vi "MAIN PROVVISORIO.vi"() -> ()   [LabVIEW 2019]
uses:
  <vilib>/DAQmx/configure/timing.llb/DAQmx Timing (Sample Clock).vi
  <vilib>/DAQmx/create/channels.llb/DAQmx Create Channel (CI-Count Edges).vi
  <vilib>/DAQmx/read.llb/DAQmx Read (Counter 1D U32 1Chan NSamp).vi
  <vilib>/DAQmx/read.llb/DAQmx Read (Analog 1D Wfm NChan NSamp).vi
  <vilib>/DAQmx/read.llb/DAQmx Read (Counter 1D DBL 1Chan NSamp).vi
  <vilib>/DAQmx/create/channels.llb/DAQmx Create Channel (AI-Voltage-Basic).vi
  <vilib>/DAQmx/create/channels.llb/DAQmx Create Channel (CI-Frequency).vi
  <vilib>/DAQmx/configure/timing.llb/DAQmx Timing (Implicit).vi
  <vilib>/Analysis/NI_AALBase.lvlib
  <vilib>/Analysis/baseanly.llb/Mean (DBL).vi
  <resource>/objmgr/daqmx.rc
  TypeDef/MISURE WT.ctl
panel:
  in  "divisor":u32=4
  in  "Tab Control":T1(tab)
  out "MISURE DA WATTMETRO":T2
  out "Waveform Chart":waveform(dbl)[](graph)
  in  "Pause Button":bool
  out "x-y":u32
  out "size(s)":i32
  in  "Initial Count":u32(ring)
  in  "Count Direction":i32(ring)=10128 items=["Count Up"=10128, "Count Down"=10124, "Externally Controlled"=10326]
  in  "Edge":i32(ring)=10280 items=["Rising"=10280, "Falling"=10171]
  in  "Analog Channel":tag="MOMENTIVEMod2/ai0:1"
  in  "Counter Input - Frequency":tag="MOMENTIVEMod1/ctr0"
  in  "Counter Input - Count Edges":tag="MOMENTIVEMod1/ctr2"
  in  "Counter Input - Count Edges Terminal":tag="/MOMENTIVEMod1/PFI0"
  in  "CI.Freq.Term":tag="/MOMENTIVEMod1/PFI1"
  in  "Rate":dbl=10000.0 format="%0.2f"
  in  "Samples per channel":i32=2000
  out "error out":errorcluster
  out "error out 2":errorcluster
  out "error out 3":errorcluster
  out "error out 4":errorcluster
  out "error out 5":errorcluster
  out "error out 6":errorcluster
  in  "Fondoscala NM":dbl=500.0
  out "COPPIA [NM]":dbl
  out "Speed [RPM]":dbl format="%#.6f"
  out "P[kW]":dbl
  in  "OFFSET NM":dbl
  in  "stop":bool
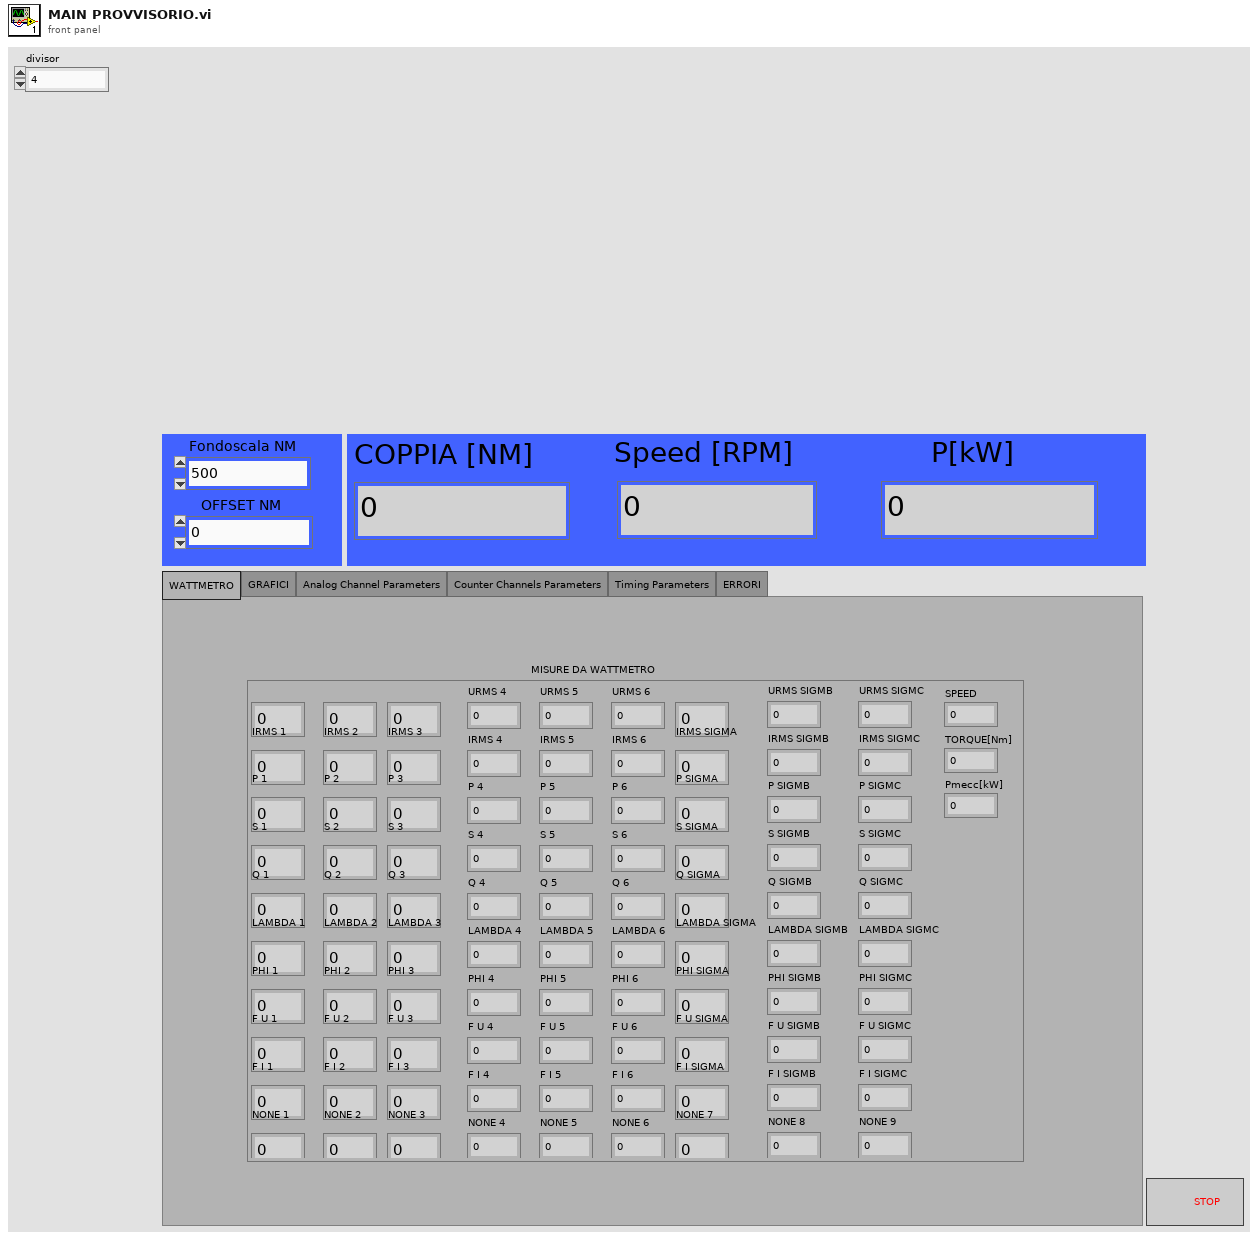
[diagram p1: front panel]
types:
  T1 = enum32{"WATTMETRO", "GRAFICI", "Analog Channel Parameters", "Counter Channels Parameters", "Timing Parameters", "ERRORI"}
  T2 = typedef "MISURE WT.ctl" = cluster{"URMS 1":dbl, "IRMS 1":dbl, "P 1":dbl, "S 1":dbl, "Q 1":dbl, "LAMBDA 1":dbl, "PHI 1":dbl, "F U 1":dbl, "F I 1":dbl, "NONE 1":dbl, "URMS 2":dbl, "IRMS 2":dbl, "P 2":dbl, "S 2":dbl, "Q 2":dbl, "LAMBDA 2":dbl, "PHI 2":dbl, "F U 2":dbl, "F I 2":dbl, "NONE 2":dbl, "URMS 3":dbl, "IRMS 3":dbl, "P 3":dbl, "S 3":dbl, "Q 3":dbl, "LAMBDA 3":dbl, "PHI 3":dbl, "F U 3":dbl, "F I 3":dbl, "NONE 3":dbl, "URMS 4":dbl, "IRMS 4":dbl, "P 4":dbl, "S 4":dbl, "Q 4":dbl, "LAMBDA 4":dbl, "PHI 4":dbl, "F U 4":dbl, "F I 4":dbl, "NONE 4":dbl, "URMS 5":dbl, "IRMS 5":dbl, "P 5":dbl, "S 5":dbl, "Q 5":dbl, "LAMBDA 5":dbl, "PHI 5":dbl, "F U 5":dbl, "F I 5":dbl, "NONE 5":dbl, "URMS 6":dbl, "IRMS 6":dbl, "P 6":dbl, "S 6":dbl, "Q 6":dbl, "LAMBDA 6":dbl, "PHI 6":dbl, "F U 6":dbl, "F I 6":dbl, "NONE 6":dbl, "URMS SIGMA":dbl, "IRMS SIGMA":dbl, "P SIGMA":dbl, "S SIGMA":dbl, "Q SIGMA":dbl, "LAMBDA SIGMA":dbl, "PHI SIGMA":dbl, "F U SIGMA":dbl, "F I SIGMA":dbl, "NONE 7":dbl, "URMS SIGMB":dbl, "IRMS SIGMB":dbl, "P SIGMB":dbl, "S SIGMB":dbl, "Q SIGMB":dbl, "LAMBDA SIGMB":dbl, "PHI SIGMB":dbl, "F U SIGMB":dbl, "F I SIGMB":dbl, "NONE 8":dbl, "URMS SIGMC":dbl, "IRMS SIGMC":dbl, "P SIGMC":dbl, "S SIGMC":dbl, "Q SIGMC":dbl, "LAMBDA SIGMC":dbl, "PHI SIGMC":dbl, "F U SIGMC":dbl, "F I SIGMC":dbl, "NONE 9":dbl, "SPEED":dbl, "TORQUE[Nm]":dbl, "Pmecc[kW]":dbl}
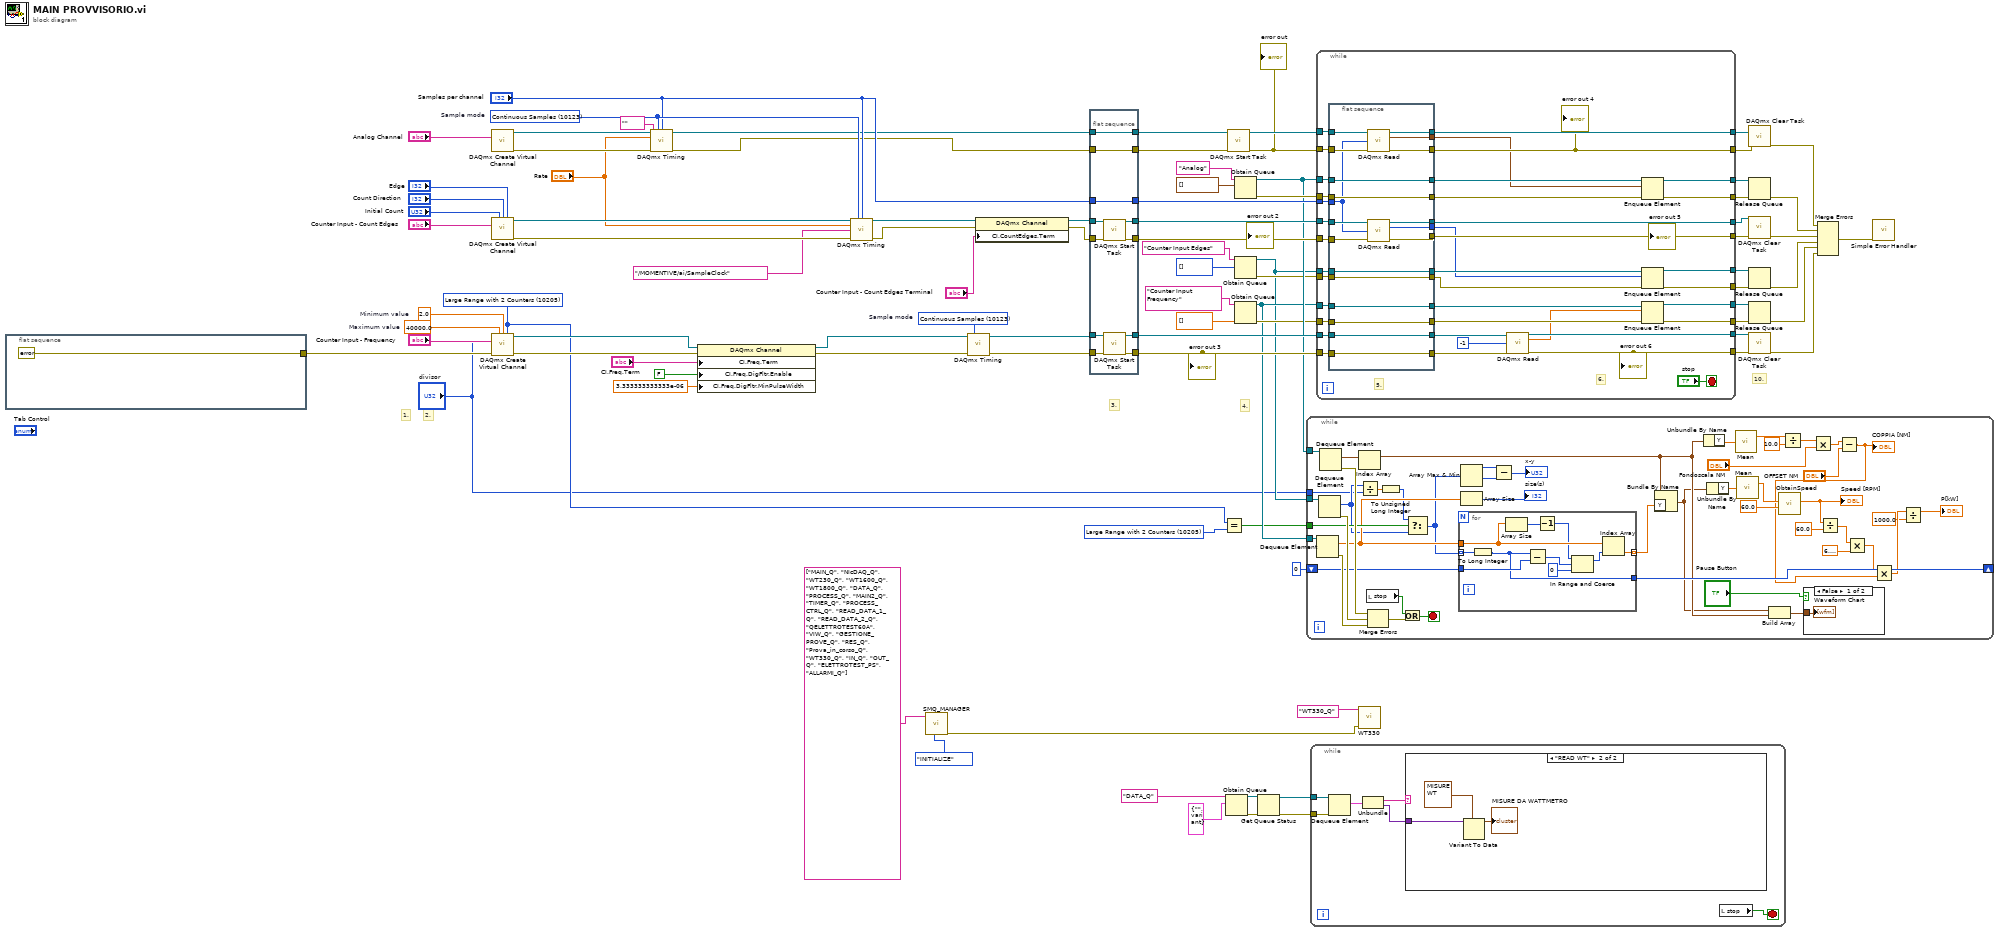
[diagram p0: block diagram]
diagram:
  w13 = 10205 items=["Low Frequency with 1 Counter"=10105, "High Frequency with 2 Counters"=10157, "Large Range with 2 Counters"=10205, "Dynamic Averaging"=16065] ("measurement method")
  w14 = 10205 items=["Low Frequency with 1 Counter"=10105, "High Frequency with 2 Counters"=10157, "Large Range with 2 Counters"=10205, "Dynamic Averaging"=16065] ("measurement method")
  w59 = 40000.0  # Maximum value
  w58 = 2.0  # Minimum value
  w60 = 10123 items=["Finite Samples"=10178, "Continuous Samples"=10123, "Hardware Timed Single Point"=12522]  # Sample mode
  w72 = 10123 items=["Finite Samples"=10178, "Continuous Samples"=10123, "Hardware Timed Single Point"=12522]  # Sample mode
  # "10."
  # "4."
  # "3."
  # "2."
  # "1."
  n1 = flat-sequence {
    tunnel: [errorcluster {"status"=FALSE, "code"=0, "source"=""} ("error constant")] -> w30
    frame #0 {
    }
  }
  n2 = call-poly <vilib>:"DAQmx Create Virtual Channel.vi"("physical channels"="Analog Channel") -> ("task out"=w83:refnum<k21>, "error out"=w82:errorcluster)  [unwired: 8 in, 5 out]
  n3 = call-poly <vilib>:"DAQmx Create Virtual Channel.vi"("initial count"="Initial Count", "count direction"="Count Direction", "edge"="Edge", "counter"="Counter Input - Count Edges") -> ("task out"=w84:refnum<k21>, "error out"=w76:errorcluster)  [unwired: 3 in, 7 out]
  n4 = call-poly <vilib>:"DAQmx Create Virtual Channel.vi"("maximum value"=w59, "minimum value"=w58, "measurement method"=w14, "counter"="Counter Input - Frequency", "divisor"="divisor", "error in"=w30) -> ("task out"=w23:refnum<k21>, "error out"=w21:errorcluster)  [unwired: 6 in, 2 out]
  n5 = call-poly <vilib>:"DAQmx Timing.vi"("task/channels in"=w83, "sample mode"=w72, "samples per channel"="Samples per channel", "rate"="Rate", "source"=tag "", "error in"=w82) -> ("task out"=w16:refnum<k21>, "error out"=w18:errorcluster)  [unwired: 1 in, 7 out]
  n6 = property class="DAQmx Channel"(reference=w23, error in=w21, "CI.Freq.Term"="CI.Freq.Term", "CI.Freq.DigFltr.Enable"=FALSE ("DI.DigFltr.Enable"), "CI.Freq.DigFltr.MinPulseWidth"=3.333333333333e-06 ("DI.DigFltr.MinPulseWidth")) -> (reference out=w22:refnum<k21>, error out=w20:errorcluster)
  n7 = call-poly <vilib>:"DAQmx Timing.vi"("task/channels in"=w84, "sample mode"=w72, "samples per channel"="Samples per channel", "rate"="Rate", "source"=tag "/MOMENTIVE/ai/SampleClock", "error in"=w76) -> ("task out"=w29:refnum<k21>, "error out"=w68:errorcluster)  [unwired: 1 in, 7 out]
  n8 = call <userlib>:"SMQ_MANAGER.vi"("Function"=enum16{"INITIALIZE", "ENQUEUE", "STOP ALL"}."INITIALIZE", "Queue array"=string[] ["MAIN_Q", "NIcDAQ_Q", "WT230_Q", "WT1600_Q", "WT1800_Q", "DATA_Q", "PROCESS_Q", "MAIN2_Q", "TIMER_Q", "PROCESS_CTRL_Q", "READ_DATA_1_Q", "READ_DATA_2_Q", "QELETTROTEST60A", "VIW_Q", "GESTIONE_PROVE_Q", "RES_Q", "Prova_in_corso_Q", "WT330_Q", "IN_Q", "OUT_Q", "ELETTROTEST_PS", "ALLARMI_Q"]) -> ("error out"=w7:errorcluster)  [unwired: 9 in]
  n9 = call-poly <vilib>:"DAQmx Timing.vi"("task/channels in"=w22, "sample mode"=w60, "error in"=w20) -> ("task out"=w27:refnum<k21>, "error out"=w28:errorcluster)  [unwired: 4 in, 7 out]
  n10 = property class="DAQmx Channel"(reference=w29, error in=w68, "CI.CountEdges.Term"="Counter Input - Count Edges Terminal") -> (reference out=w70:refnum<k21>, error out=w69:errorcluster)
  n11 = flat-sequence {
    tunnel: [w102] -> w75
    tunnel: [w101] -> w71
    tunnel: w70 -> [w100]
    tunnel: w69 -> [w99]
    tunnel: w27 -> [w98]
    tunnel: w28 -> [w97]
    tunnel: w16 -> [w96]
    tunnel: [w96] -> w66
    tunnel: [w95] -> w65
    tunnel: w18 -> [w95]
    tunnel: [w94] -> w64
    tunnel: [w93] -> w63
    tunnel: "Samples per channel" -> [w92]
    tunnel: [w92] -> w55
    frame #0 {
      n12 = call <vilib>:"DAQmx Start Task.vi"("task/channels in"=w100, "error in"=w99) -> ("task out"=w102:refnum<k21>, "error out"=w101:errorcluster)  [unwired: 12 out]
      n13 = call <vilib>:"DAQmx Start Task.vi"("task/channels in"=w98, "error in"=w97) -> ("task out"=w94:refnum<k21>, "error out"=w93:errorcluster)  [unwired: 12 out]
    }
  }
  n14 = Equal?(x=w14, y=w13) -> (x = y?=w12:bool)
  n15 = Obtain Queue(name (unnamed)="DATA_Q" ("Queue Name"), element data type=cluster{"String":string, "variant":variant} {"String"="", "variant"=variant} ("element")) -> (queue out=w4:refnum<queue>, error out=w3:errorcluster)  [unwired: 3 in, 1 out]
  n16 = call <vilib>:"DAQmx Start Task.vi"("task/channels in"=w66, "error in"=w65) -> ("task out"=w81:refnum<k21>, "error out"=w80:errorcluster)  [unwired: 12 out]
  "error out" <- w80
  n17 = Obtain Queue(name (unnamed)="Analog", element data type=waveform(dbl)[] [] ("data")) -> (queue out=w47:refnum<queue>, error out=w52:errorcluster)  [unwired: 3 in, 1 out]
  n18 = Obtain Queue(name (unnamed)="Counter Input Edges", element data type=u32[] [] ("data")) -> (queue out=w33:refnum<queue>, error out=w39:errorcluster)  [unwired: 3 in, 1 out]
  n19 = Obtain Queue(name (unnamed)="Counter Input Frequency", element data type=dbl[] [] ("data")) -> (queue out=w41:refnum<queue>, error out=w43:errorcluster)  [unwired: 3 in, 1 out]
  n20 = Get Queue Status(queue=w4, error in (no error)=w3) -> (queue out=w2:refnum<queue>, error out=w1:errorcluster)  [unwired: 1 in, 6 out]
  n21 = while {
    tunnel: w47 -> [w149]
    tunnel: w41 -> [w148]
    tunnel: w33 -> [w147]
    shift-right: [w138] -> _
    shift-left: 0 -> [w139]
    tunnel: w12 -> [w137]
    tunnel: "divisor" -> [w128]
    stop <- w104 stop-if-true
    n22 = Dequeue Element(queue=w148) -> (element=w133:dbl[], error out=w143:errorcluster)  [unwired: 2 in, 2 out]
    n23 = Dequeue Element(queue=w147) -> (element=w130:u32[], error out=w144:errorcluster)  [unwired: 2 in, 2 out]
    n24 = Dequeue Element(queue=w149) -> (element=w142:waveform(dbl)[], error out=w145:errorcluster)  [unwired: 2 in, 2 out]
    n25 = Index Array(array=w142) -> (element=w126:waveform(dbl))  [unwired: 1 in]
    n26 = Divide(x=w130, y=w128) -> (x/y=w129:dbl[])
    n27 = local read "stop"() -> (w103:bool)
    n28 = Merge Errors(w145, w144, w143) -> (w146:errorcluster)
    n29 = To Unsigned Long Integer(number=w129) -> (unsigned 32bit integer=w127:u32[])
    n30 = Or(x=w103, y=w146) -> (x .or. y?=w104:bool)
    n31 = Select(t=w127, s=w137, f=w130) -> (s? t:f=w131:u32[])
    n32 = for {
      tunnel: w131 -> [w159] mode=indexing
      tunnel: w133 -> [w156]
      tunnel: [w160] -> w141 mode=indexing
      tunnel: w139 -> [w158]
      tunnel: [w157] -> w138
      n33 = To Long Integer(number=w159) -> (32bit integer=w157:i32)
      n34 = Array Size(array=w156) -> (size(s)=w152:i32)
      n35 = Subtract(x=w157, y=w158) -> (x-y=w155:i32)
      n36 = Decrement(x=w152) -> (x-1=w151:i32)
      n37 = In Range and Coerce(upper limit=w151, x=w155, lower limit=0) -> (coerced(x)=w153:i32)  [unwired: 1 out]
      n38 = Index Array(array=w156, index=w153) -> (element=w160:dbl)
    }
    n39 = Array Max & Min(array=w131) -> (max value=w136:u32, min value=w135:u32)  [unwired: 2 out]
    n40 = Array Size(array=w133) -> (size(s)=→"size(s)":i32)
    n41 = Subtract(x=w136, y=w135) -> (x-y=→"x-y":u32)
    n42 = Bundle By Name(cluster=w126, "Y"=w141) -> (w125:waveform(dbl))
    n43 = Unbundle By Name(w126) -> ("Y"=w124:dbl[])
    n44 = Unbundle By Name(w125) -> ("Y"=w123:dbl[])
    n45 = call-poly <vilib>:"Mean.vi"("X"=w124) -> ("mean"=w122:dbl)  [unwired: 1 out]
    n46 = call-poly <vilib>:"Mean.vi"("X"=w123) -> ("mean"=w118:dbl)  [unwired: 1 out]
    n47 = Build Array(w125, w126) -> (w140:waveform(dbl)[])
    n48 = call "ObtainSpeed.vi"("Pulses per Revolution"=60.0, "Counter Frequency"=w118) -> ("Speed [RPM]"=w112:dbl)  [unwired: 7 in, 2 out]
    "Speed [RPM]" <- w112
    n49 = Divide(x=w122, y=10.0) -> (x/y=w120:dbl)
    n50 = case shown="False" "Pause Button" {
      tunnel: w140 -> [w150 _]
      frame False {
        "Waveform Chart" <- w150
      }
      frame True {
      }
    }
    n51 = Multiply(x=w120, y="Fondoscala NM") -> (x*y=w107:dbl)
    n52 = Divide(x=w112, y=60.0) -> (x/y=w114:dbl)
    n53 = Subtract(x=w107, y="OFFSET NM") -> (x-y=w105:dbl)
    "COPPIA [NM]" <- w105
    n54 = Multiply(x=w114, y=6.283185307179586) -> (x*y=w116:dbl)
    n55 = Multiply(x=w116, y=w105) -> (x*y=w111:dbl)
    n56 = Divide(x=w111, y=1000.0) -> (x/y=→"P[kW]":dbl)
  }
  n57 = while {
    tunnel: w2 -> [w165]
    tunnel: w1 -> [w164]
    stop <- w163 stop-if-true
    n58 = Dequeue Element(queue=w165, error in (no error)=w164) -> (element=w166:cluster{"String":string, "variant":variant})  [unwired: 1 in, 3 out]
    n59 = Unbundle(w166) -> ("String"=w162:string, "variant"=w161:variant)
    n60 = case shown="\"READ WT\"" w162 {
      tunnel: w161 -> [_ w169]
      frame "False", Default {
      }
      frame "READ WT" {
        n61 = Variant To Data(type=T2 {"URMS 1"=0.0, "IRMS 1"=0.0, "P 1"=0.0, "S 1"=0.0, "Q 1"=0.0, "LAMBDA 1"=0.0, "PHI 1"=0.0, "F U 1"=0.0, "F I 1"=0.0, "NONE 1"=0.0, "URMS 2"=0.0, "IRMS 2"=0.0, "P 2"=0.0, "S 2"=0.0, "Q 2"=0.0, "LAMBDA 2"=0.0, "PHI 2"=0.0, "F U 2"=0.0, "F I 2"=0.0, "NONE 2"=0.0, "URMS 3"=0.0, "IRMS 3"=0.0, "P 3"=0.0, "S 3"=0.0, "Q 3"=0.0, "LAMBDA 3"=0.0, "PHI 3"=0.0, "F U 3"=0.0, "F I 3"=0.0, "NONE 3"=0.0, "URMS 4"=0.0, "IRMS 4"=0.0, "P 4"=0.0, "S 4"=0.0, "Q 4"=0.0, "LAMBDA 4"=0.0, "PHI 4"=0.0, "F U 4"=0.0, "F I 4"=0.0, "NONE 4"=0.0, "URMS 5"=0.0, "IRMS 5"=0.0, "P 5"=0.0, "S 5"=0.0, "Q 5"=0.0, "LAMBDA 5"=0.0, "PHI 5"=0.0, "F U 5"=0.0, "F I 5"=0.0, "NONE 5"=0.0, "URMS 6"=0.0, "IRMS 6"=0.0, "P 6"=0.0, "S 6"=0.0, "Q 6"=0.0, "LAMBDA 6"=0.0, "PHI 6"=0.0, "F U 6"=0.0, "F I 6"=0.0, "NONE 6"=0.0, "URMS SIGMA"=0.0, "IRMS SIGMA"=0.0, "P SIGMA"=0.0, "S SIGMA"=0.0, "Q SIGMA"=0.0, "LAMBDA SIGMA"=0.0, "PHI SIGMA"=0.0, "F U SIGMA"=0.0, "F I SIGMA"=0.0, "NONE 7"=0.0, "URMS SIGMB"=0.0, "IRMS SIGMB"=0.0, "P SIGMB"=0.0, "S SIGMB"=0.0, "Q SIGMB"=0.0, "LAMBDA SIGMB"=0.0, "PHI SIGMB"=0.0, "F U SIGMB"=0.0, "F I SIGMB"=0.0, "NONE 8"=0.0, "URMS SIGMC"=0.0, "IRMS SIGMC"=0.0, "P SIGMC"=0.0, "S SIGMC"=0.0, "Q SIGMC"=0.0, "LAMBDA SIGMC"=0.0, "PHI SIGMC"=0.0, "F U SIGMC"=0.0, "F I SIGMC"=0.0, "NONE 9"=0.0, "SPEED"=0.0, "TORQUE[Nm]"=0.0, "Pmecc[kW]"=0.0} ("MISURE WT"), Variant=w169) -> (data=→"MISURE DA WATTMETRO":T2)  [unwired: 1 in, 1 out]
      }
    }
    n62 = local read "stop"() -> (w163:bool)
  }
  n63 = while {
    tunnel: w71 -> [w207]
    tunnel: w75 -> [w206]
    tunnel: [w205] -> w90
    tunnel: [w198] -> w85
    tunnel: w81 -> [w203]
    tunnel: w80 -> [w204]
    tunnel: [w201] -> w79
    tunnel: [w202] -> w78
    tunnel: w64 -> [w197]
    tunnel: w63 -> [w196]
    tunnel: [w200] -> w62
    tunnel: [w199] -> w61
    tunnel: w55 -> [w192]
    tunnel: w47 -> [w191]
    tunnel: w52 -> [w190]
    tunnel: [w186] -> w51
    tunnel: [w185] -> w50
    tunnel: w41 -> [w184]
    tunnel: [w182] -> w44
    tunnel: w43 -> [w181]
    tunnel: [w179] -> w42
    tunnel: w33 -> [w178]
    tunnel: w39 -> [w176]
    tunnel: [w173] -> w38
    tunnel: [w172] -> w37
    stop <- "stop" stop-if-true
    # "6."
    # "5."
    n64 = flat-sequence {
      tunnel: w207 -> [w226]
      tunnel: w206 -> [w225]
      tunnel: [w224] -> w205
      tunnel: w204 -> [w223]
      tunnel: w203 -> [w222]
      tunnel: [w221] -> w202
      tunnel: [w220] -> w201
      tunnel: [w219] -> w174
      tunnel: [w209] -> w187
      tunnel: [w218] -> w198
      tunnel: w197 -> [w216]
      tunnel: w196 -> [w217]
      tunnel: [w217] -> w195
      tunnel: [w216] -> w194
      tunnel: w192 -> [w208]
      tunnel: w191 -> [w215]
      tunnel: w190 -> [w214]
      tunnel: [w215] -> w189
      tunnel: [w214] -> w188
      tunnel: w184 -> [w213]
      tunnel: [w213] -> w183
      tunnel: w181 -> [w212]
      tunnel: [w212] -> w180
      tunnel: w178 -> [w210]
      tunnel: [w210] -> w177
      tunnel: w176 -> [w211]
      tunnel: [w211] -> w175
      frame #0 {
        n65 = call-poly <vilib>:"DAQmx Read.vi"("task/channels in"=w222, "number of samples per channel"=w208, "error in"=w223) -> ("task out"=w221:refnum<k21>, "data"=w209:waveform(dbl)[], "error out"=w220:errorcluster)  [unwired: 10 out]
        n66 = call-poly <vilib>:"DAQmx Read.vi"("task/channels in"=w225, "number of samples per channel"=w208, "error in"=w226) -> ("task out"=w224:refnum<k21>, "data"=w219:u32[], "error out"=w218:errorcluster)  [unwired: 10 out]
      }
    }
    n67 = call-poly <vilib>:"DAQmx Read.vi"("task/channels in"=w194, "number of samples per channel"=-1, "error in"=w195) -> ("task out"=w200:refnum<k21>, "data"=w171:dbl[], "error out"=w199:errorcluster)  [unwired: 10 out]
    "error out 6" <- w199
    n68 = Enqueue Element(queue=w189, element=w187, error in (no error)=w188) -> (queue out=w186:refnum<queue>, error out=w185:errorcluster)  [unwired: 1 in, 1 out]
    n69 = Enqueue Element(queue=w177, element=w174, error in (no error)=w175) -> (queue out=w173:refnum<queue>, error out=w172:errorcluster)  [unwired: 1 in, 1 out]
    n70 = Enqueue Element(queue=w183, element=w171, error in (no error)=w180) -> (queue out=w182:refnum<queue>, error out=w179:errorcluster)  [unwired: 1 in, 1 out]
    "error out 4" <- w201
    "error out 5" <- w198
  }
  n71 = call "WT330.vi"("error in (no error)"=w7, "Queue Name"="WT330_Q") -> ()  [unwired: 8 in, 2 out]
  n72 = call <vilib>:"DAQmx Clear Task.vi"("task in"=w78, "error in"=w79) -> ("error out"=w49:errorcluster)  [unwired: 13 out]
  n73 = Release Queue(queue=w51, error in (no error)=w50) -> (error out=w48:errorcluster)  [unwired: 1 in, 2 out]
  n74 = call <vilib>:"DAQmx Clear Task.vi"("task in"=w90, "error in"=w85) -> ("error out"=w73:errorcluster)  [unwired: 13 out]
  n75 = Release Queue(queue=w38, error in (no error)=w37) -> (error out=w34:errorcluster)  [unwired: 1 in, 2 out]
  n76 = Release Queue(queue=w44, error in (no error)=w42) -> (error out=w35:errorcluster)  [unwired: 1 in, 2 out]
  n77 = call <vilib>:"DAQmx Clear Task.vi"("task in"=w62, "error in"=w61) -> ("error out"=w36:errorcluster)  [unwired: 13 out]
  n78 = Merge Errors(w49, w48, w73, w34, w35, w36) -> (w74:errorcluster)
  n79 = call <vilib>:"Simple Error Handler.vi"("error in (no error)"=w74) -> ()  [unwired: 1 in, 8 out]
  "error out 2" <- w71
  "error out 3" <- w63
